vi "Untitled 2.vi"() -> ()   [LabVIEW 2018]
uses:
  Source/Image/Image Process.lvclass
panel:
  in  "Rectangle 2":T1
  out "Image 2":T2(plugin-control)
  out "Image":T2(plugin-control)
  out "new picture":picture
  out "Rectangle":T1
  in  "threshold":u8=10
  out "error out":errorcluster
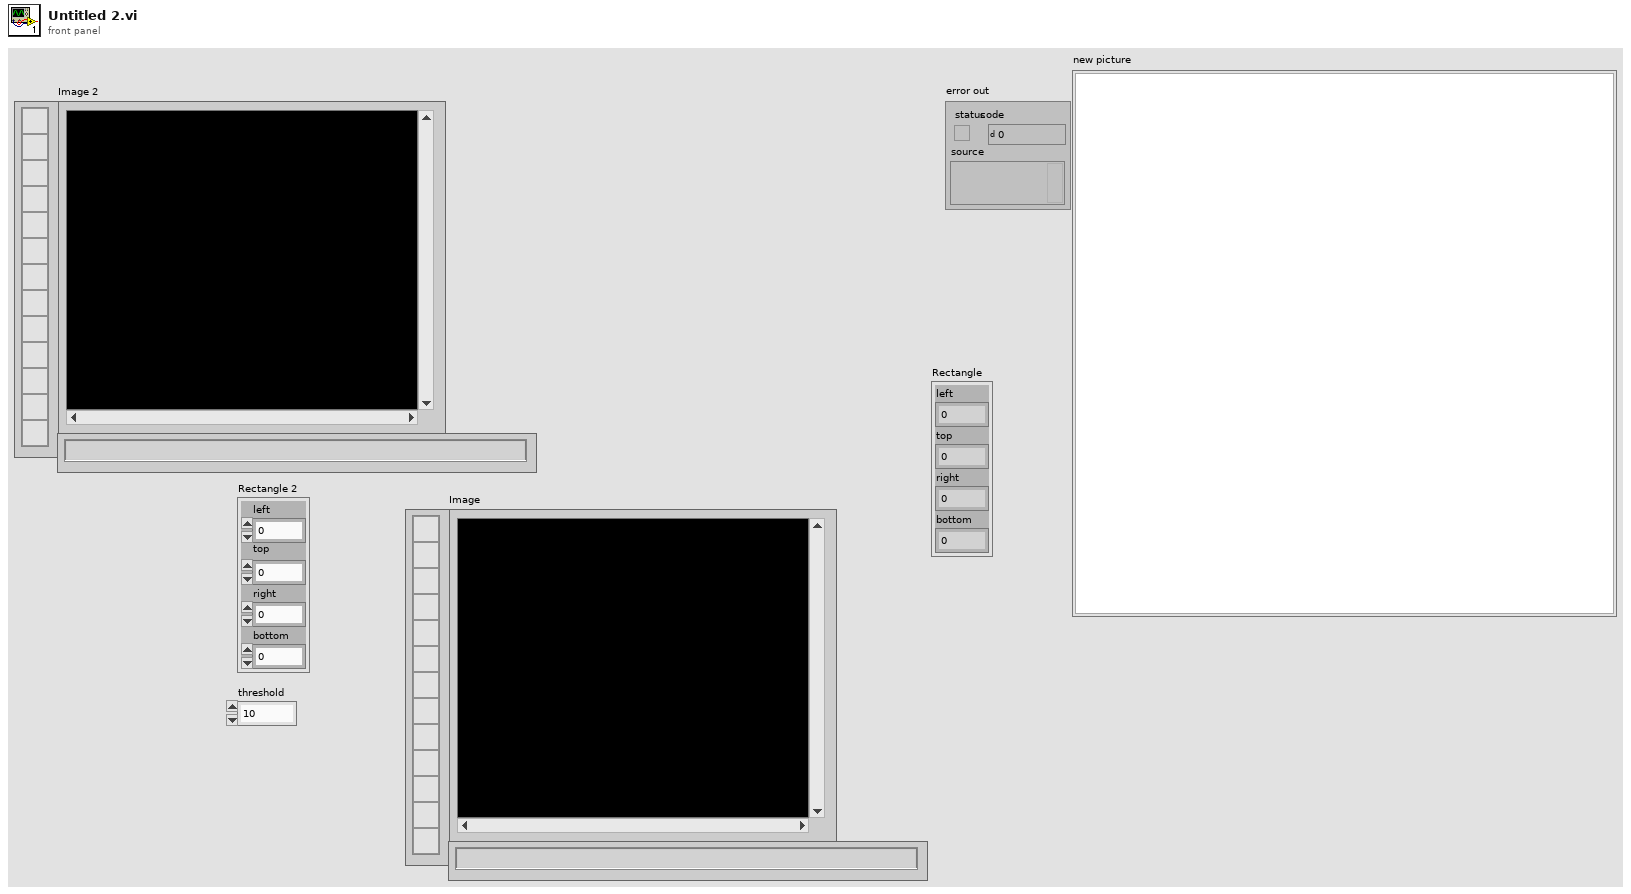
[diagram p1: front panel]
types:
  T1 = cluster{"left":i16, "top":i16, "right":i16, "bottom":i16}
  T2 = typedef "IMAQ Image.ctl" = refnum<image>
  T3 = typedef "Image Type" = u32
  T4 = typedef "imagedata.ctl" = cluster{"image type":i32, "image depth":i32, "image":u8[], "mask":u8[], "colors":u32[], "Rectangle":cluster{"left":i16, "top":i16, "right":i16, "bottom":i16}}
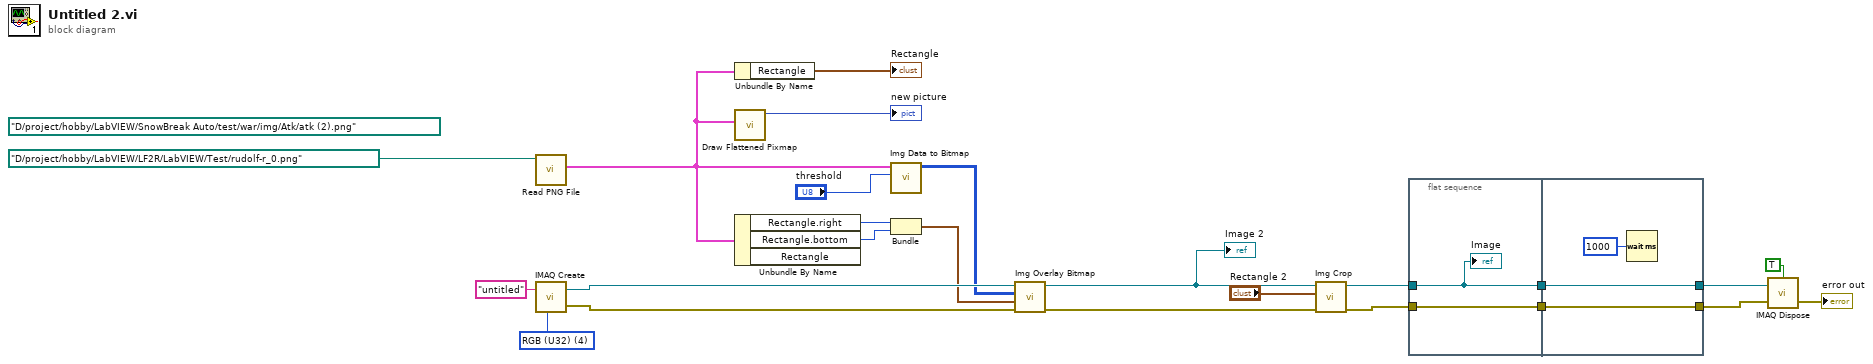
[diagram p0: block diagram]
diagram:
  (unwired) path "D:/project/hobby/LabVIEW/SnowBreak Auto/test/war/img/Atk/atk (2).png" ("path to PNG file")
  w23 = T3 4 items=["Grayscale (U8)", "Grayscale (I16)", "Grayscale (SGL)", "Complex (CSG)", "RGB (U32)", "HSL (U32)", "RGB (U64)", "Grayscale (U16)"] ("Image Type")
  n1 = call <vilib>:"Read PNG File.vi"("path to PNG file"=path "D:/project/hobby/LabVIEW/LF2R/LabVIEW/Test/rudolf-r_0.png") -> ("image data"=w11:T4)  [unwired: 8 in, 2 out]
  n2 = call "IMAQ Create"("Image Name"="untitled", "Image Type"=w23) -> ("New Image"=w9:T2, "error out"=w8:errorcluster)  [unwired: 3 in]
  n3 = Unbundle By Name(w11) -> ("Rectangle"=→"Rectangle":T1)
  n4 = call <vilib>:"Draw Flattened Pixmap.vi"("image data"=w11) -> ("new picture"=→"new picture":picture)  [unwired: 8 in]
  n5 = Unbundle By Name(w11) -> ("Rectangle.right"=w6:i16, "Rectangle.bottom"=w5:i16)  [unwired: 1 out]
  n6 = call "Img Data to Bitmap.vi"("threshold"="threshold", "image data"=w11) -> ("bitmap"=w7:u32[][])  [unwired: 9 in]
  n7 = Bundle("right"=w6, "bottom"=w5) -> (w4:cluster{"right":i16, "bottom":i16})  [unwired: 1 in]
  n8 = call "Img Overlay Bitmap.vi"("error in (no error)"=w8, "Size"=w4, "Bitmap"=w7, "Image"=w9) -> ("error out"=w3:errorcluster, "Image Out"=w2:T2)  [unwired: 6 in]
  "Image 2" <- w2
  n9 = call "Img Crop.vi"("error in (no error)"=w3, "Rectangle"="Rectangle 2", "Image Src"=w2) -> ("error out"=w17:errorcluster, "Image Out"=w19:T2)  [unwired: 7 in]
  n10 = flat-sequence {
    tunnel: w19 -> [w25]
    tunnel: w17 -> [w26]
    tunnel: [w25] -> w15
    tunnel: [w26] -> w14
    tunnel: [w28] -> w16
    tunnel: [w29] -> w18
    tunnel: w15 -> [w29]
    tunnel: w14 -> [w28]
    frame #0 {
      "Image" <- w25
    }
    frame #1 {
      n11 = Wait (ms)(milliseconds to wait=u32 1000) -> ()  [unwired: 1 out]
    }
  }
  n12 = call "IMAQ Dispose"("All Images? (No)"=TRUE, "Image"=w18, "error in (no error)"=w16) -> ("error out"=→"error out":errorcluster)  [unwired: 3 in]
